vi "Log to CSV.vi"(2 "Data Str":string, 3 "error in (no error)":errorcluster, 4 "Path":path) -> (7 "error out":errorcluster)   [LabVIEW 2015]
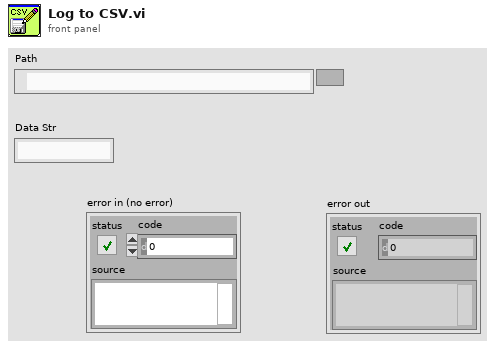
[diagram p1: front panel]
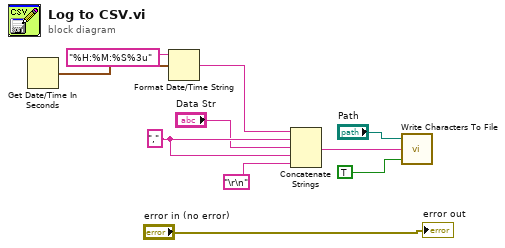
[diagram p0: block diagram]
diagram:
  w3 = ","
  n1 = Get Date/Time In Seconds() -> (seconds since 1Jan1904=w9:timestamp)
  n2 = Format Date/Time String(time format string (%c)="%H:%M:%S%3u", seconds (now)=w9) -> (date/time string=w6:string)  [unwired: 1 in]
  n3 = Concatenate Strings(w6, w3, "Data Str", w3, "\r\n") -> (w4:string)
  n4 = call <vilib>:"Write Characters To File.vi"("append to file? (new file:F)"=TRUE, "character string"=w4, "file path (dialog if empty)"="Path") -> ()  [unwired: 2 in, 1 out]
  "error out" <- "error in (no error)"
